vi "updateWaypoints.vi"(8 "error in (no error)":errorcluster, 11 "Idle in":refnum<class "Idle.lvclass">) -> (0 "error out":errorcluster, 3 "Idle out":refnum<class "Idle.lvclass">)   [LabVIEW 2011, in "Idle.lvclass"]
doc: "Updates the waypoints global variable as necessary in order to complete this mission.\n\nIn this case, no updates are needed. (Possible future improvement would be to allow this waypoint to move when the robot is under human control.)\n\nNote: This is a dynamic dispatch method of GenericMission. The correct method will be called based on the run-time class of this object, a child class of GenericMission.\n\nAuthor: Jared Kirschner"
uses:
  Idle.lvclass
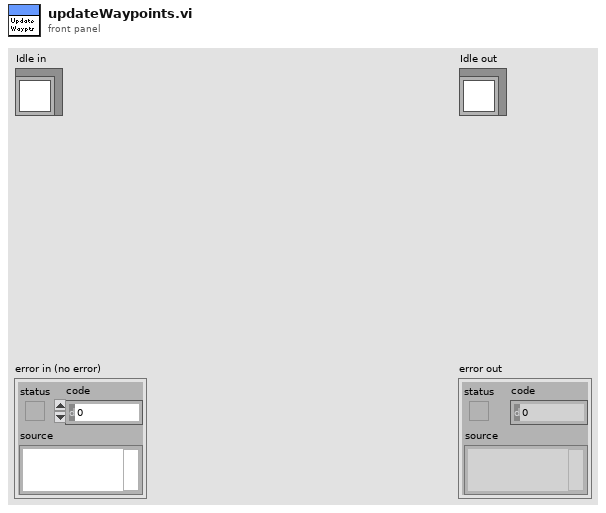
[diagram p1: front panel]
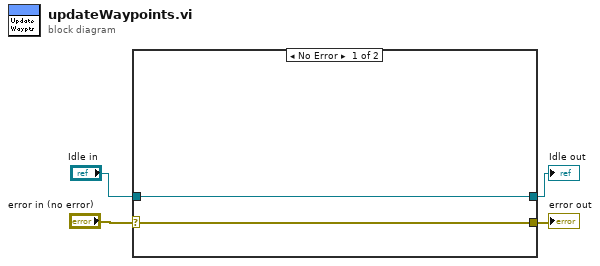
[diagram p0: block diagram]
diagram:
  n1 = case shown="No Error" "error in (no error)" {
    selector: "error in (no error)" -> [w6 w8]
    tunnel: [w6 w8] -> w3
    tunnel: "Idle in" -> [w5 w7]
    tunnel: [w5 w7] -> w1
    frame No Error {
    }
    frame Error {
    }
  }
  "error out" <- w3
  "Idle out" <- w1
